vi "archivoExcel.vi"(7 "worksheet index (0)":i32) -> (2 "opciones":bool[](array[boolean]), 4 "Control de espejos 3":T6={"Movimiento de spot en y"=0.78, "Movimiento de spot en x"=0.5255, "tipo "=enum."barrido", "yFin"=0.82, "Paso"=0.01, "xFin"=0.5655} {"Movimiento de spot en x" scale=-10.0..10.0; "Movimiento de spot en y" min=-10.0 max=10.0 scale=-10.0..10.0}, 6 "config. Polarizador 2":T5={"pos inic"=0.0, "pos.final"=5.0, "incremento"=1.0, "velocidad"=0.0}, 8 "Config. fotodiodo y potenciometro 2":T4={"tiempo. lect."=300, "num. med"=20, "tiempo. lectura"=0, "average rate"=0, "Readout Config"="POW", "Tipo de Medición"=enum."Lockin", "usar multimetro"=FALSE}, 10 "Config. voltaje y corriente 2":T3 {"Measurement Function (0:Voltage)" items=["Voltage", "Current", "Power"]; "Unit(V)" items=["V", "mV", "kV", "A", "mA"]; "Function(0:Voltage)" items=["Voltage", "Current"]}, 14 "orden 2":T1(array[ring]), 15 "Control CCD 2":T2={"Numero de lecturas"=0, "tiempo de lectura (ms)"=100, "Exposure"=0.053229, "Valor Gamma"=1.0, "Ganancia"=33, "Opción"=enum."Espectro", "VISA resource name"="", "Enable Strobe (Disabled)"=FALSE} {"Ganancia" min=0 max=100; "Valor Gamma" min=1.0 max=2.2; "Exposure" min=5e-05 max=0.053229})   [LabVIEW 2016]
uses:
  <vilib>/addons/_office/excel.llb/Excel Get Data ([str]).vi
  <vilib>/Utility/NIReport.llb/NI_report.lvclass
  <vilib>/Utility/NIReport.llb/Excel/NI_Excel.lvclass
  <vilib>/addons/_office/NI_ReportGenerationToolkit.lvlib
panel:
  out "orden":T1(array[ring])
  out "data":string[][](array[string])
  # "Espectro"
  # "Imágen"
  # "Amplificador Lock in"
  # "potenciometro"
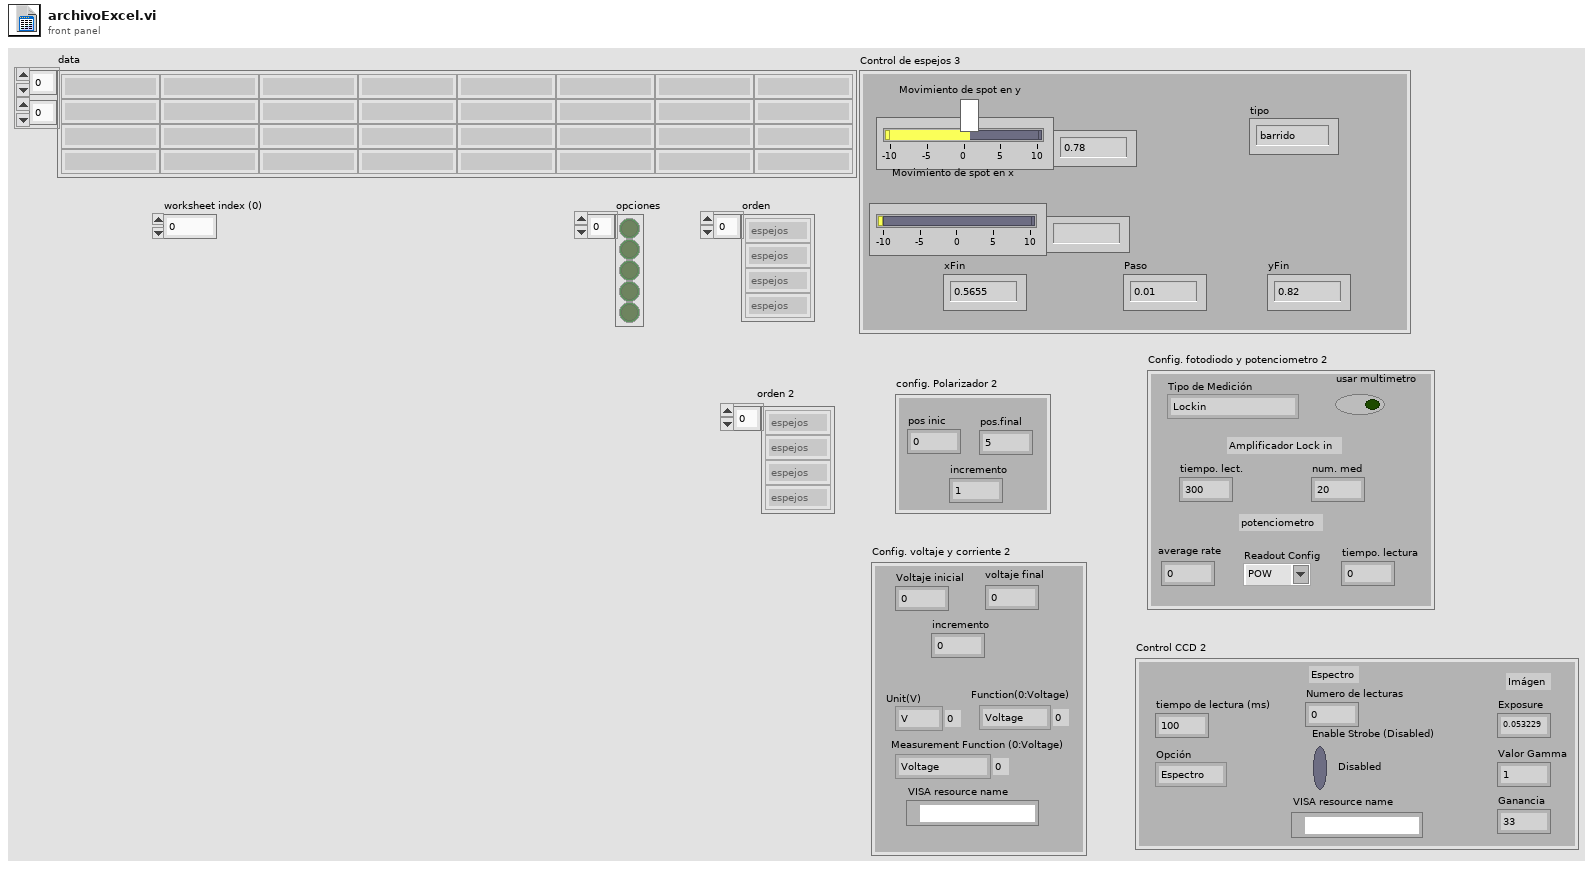
[diagram p1: front panel]
types:
  T1 = enum16{"espejos", "polarizador", "voltaje", "potenciometro y lockin", "CCD"}[]
  T2 = cluster{"Numero de lecturas":i32, "tiempo de lectura (ms)":u32, "Exposure":dbl, "Valor Gamma":dbl, "Ganancia":i64, "Opción":enum16{"Espectro", "Imágen"}, "VISA resource name":refnum<visa-resource-name>, "Enable Strobe (Disabled)":bool}
  T3 = cluster{"Voltaje inicial":dbl, "incremento":dbl, " voltaje final":dbl, "Function(0:Voltage)":u16, "Unit(V)":u16, "Measurement Function (0:Voltage)":u16, "VISA resource name":refnum<visa-resource-name>}
  T4 = cluster{"tiempo. lect.":i32, "num. med":i32, "tiempo. lectura":i32, "average rate":i32, "Readout Config":string, "Tipo de Medición":enum16{"Lockin", "Lockin-potenciometro", "Potenciometro"}, "usar multimetro":bool}
  T5 = cluster{"pos inic":dbl, "pos.final":dbl, "incremento":dbl, "velocidad":dbl}
  T6 = cluster{"Movimiento de spot en y":dbl, "Movimiento de spot en x":ext, "tipo ":enum16{"manual", "barrido"}, "yFin":dbl, "Paso":dbl, "xFin":dbl}
  T7 = enum16{"Standard Report", "HTML", "Word", "Excel"}
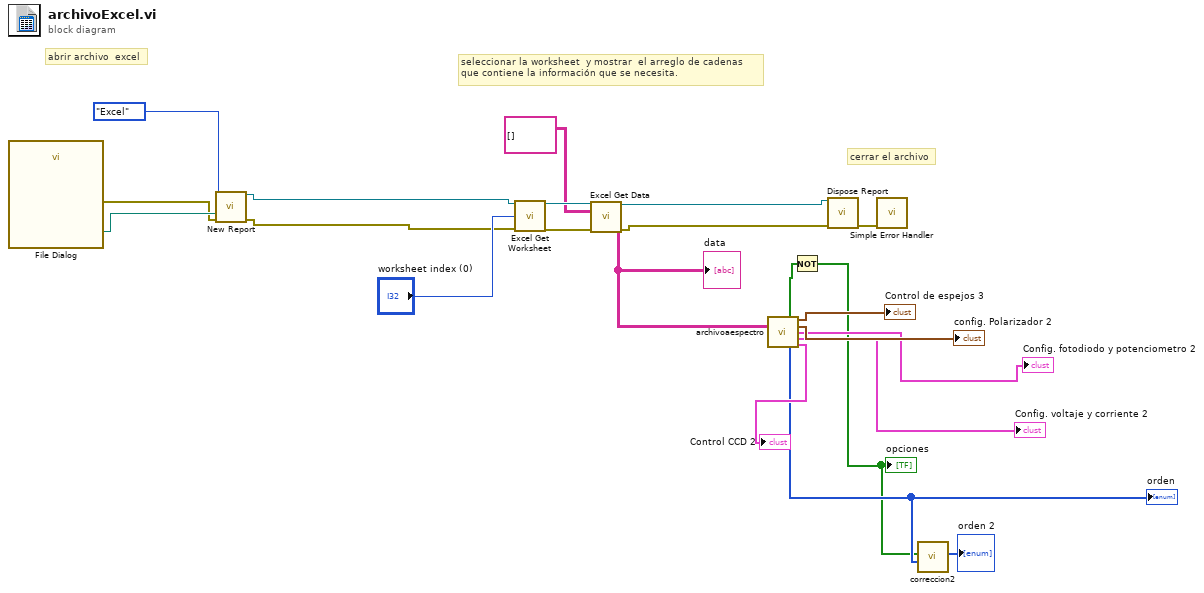
[diagram p0: block diagram]
diagram:
  # "cerrar el archivo"
  # "seleccionar la worksheet  y mostrar  el arreglo de cadenas\nque contiene la información que se necesita."
  # "abrir archivo  excel"
  n1 = call "File Dialog"() -> ("selected path"=w21:path, "error out"=w20:errorcluster)  [unwired: 12 in, 2 out]
  n2 = call <vilib>:"New Report.vi"("report type"=T7."Excel", "template (empty)"=w21, "error in (no error)"=w20) -> ("report out"=w12:refnum<class "NI_report.lvclass">, "error out"=w11:errorcluster)  [unwired: 11 in]
  n3 = call <vilib>:"Excel Get Worksheet.vi"("report in"=w12, "worksheet index (0)"="worksheet index (0)", "error in (no error)"=w11) -> ("report out"=w18:refnum<class "NI_report.lvclass">, "error out"=w17:errorcluster)  [unwired: 11 in]
  n4 = call-poly <vilib>:"Excel Get Data.vi"("report in"=w18, "data type"=string[][] [], "error in (no error)"=w17) -> ("report out"=w15:refnum<class "NI_report.lvclass">, "data"=w10:string[][], "error out"=w14:errorcluster)  [unwired: 10 in]
  "data" <- w10
  n5 = call "archivoaespectro.vi"("data 2"=w10) -> ("opciones"=w4:bool[], "Control de espejos 3"=→"Control de espejos 3":T6, "config. Polarizador 2"=→"config. Polarizador 2":T5, "Config. fotodiodo y potenciometro 2"=→"Config. fotodiodo y potenciometro 2":T4, "Config. voltaje y corriente 2"=→"Config. voltaje y corriente 2":T3, "orden"=w3:T1, "Control CCD 2"=→"Control CCD 2":T2)  [unwired: 8 in]
  "orden" <- w3
  n6 = Not(x=w4) -> (.not. x?=w2:bool[])
  "opciones" <- w2
  n7 = call-dynamic "Dispose Report.vi"("report in"=w15, "error in (no error)"=w14) -> ("error out"=w19:errorcluster)  [unwired: 13 in]
  n8 = call <vilib>:"Simple Error Handler.vi"("error in (no error)"=w19) -> ()  [unwired: 4 in, 5 out]
  n9 = call "correccion2.vi"("orden 2"=w3, "opciones"=w2) -> ("orden"=→"orden 2":T1)  [unwired: 9 in]
